vi "Get Localhost Name.vi"(8 "error in (no error)":errorcluster, 11 "Child_1 in":refnum<class "SW_Interface_Class.lvclass">) -> (0 "error out":errorcluster, 1 "PC Name":string, 3 "Child_1 out":refnum<class "SW_Interface_Class.lvclass">)   [LabVIEW 2023, in "SW_Interface_Actor.lvlib" / "SW_Interface_Class.lvclass"]
uses:
  SW_Interface_Class.lvclass
  Abstraction_Interface_Class/Abstraction_Interface_Class.lvclass
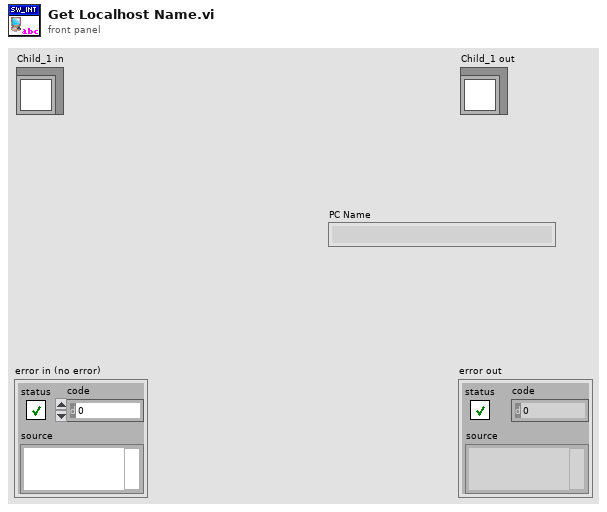
[diagram p1: front panel]
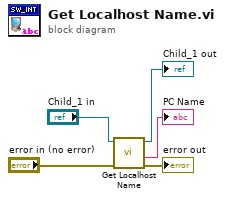
[diagram p0: block diagram]
diagram:
  n1 = call-parent "Get Localhost Name.vi"("error in (no error)"="error in (no error)", "Interface_Class in"="Child_1 in") -> ("error out"=→"error out":errorcluster, "PC Name"=→"PC Name":string, "Interface_Class out"=→"Child_1 out":refnum<class "SW_Interface_Class.lvclass">)  [unwired: 7 in]
